vi "Create PINGREQ Packet.vi"(5 "PINGREC in":refnum<class "PINGREC.lvclass">, 8 "error in (no error)":errorcluster) -> (0 "error out":errorcluster, 3 "PINGREC out":refnum<class "PINGREC.lvclass">)   [LabVIEW 2013, in "PINGREC.lvclass"]
uses:
  PINGREC.lvclass
  ControlPacket/ControlPacket.lvclass/ControlPacket.ctl
  ControlPacket/ControlPacket.lvclass
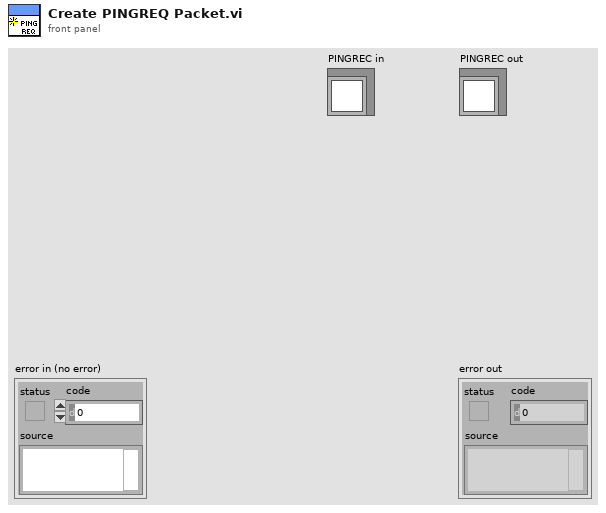
[diagram p1: front panel]
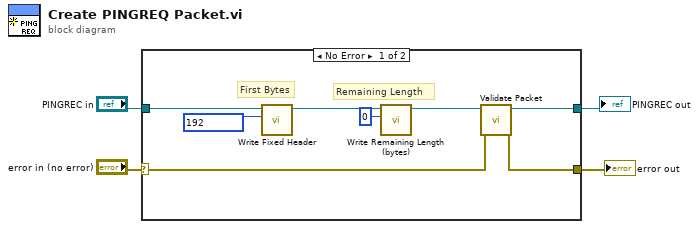
[diagram p0: block diagram]
diagram:
  n1 = case shown="No Error" "error in (no error)" {
    selector: "error in (no error)" -> [w6 w14]
    tunnel: [w5 w14] -> w1
    tunnel: [w7 w13] -> w2
    tunnel: "PINGREC in" -> [w12 w13]
    frame No Error {
      # "Remaining Length"
      # "First Bytes"
      n2 = call "Write Fixed Header.vi"("Fixed Header"=u8 192, "ControlPacket in"=w12) -> ("ControlPacket out"=w11:refnum<class "PINGREC.lvclass">)  [unwired: 9 in]
      n3 = call "Write Remaining Length (bytes).vi"("Remaining Length (bytes)"=u32 0, "ControlPacket in"=w11) -> ("ControlPacket out"=w8:refnum<class "PINGREC.lvclass">)  [unwired: 9 in]
      n4 = call "Validate Packet.vi"("error in (no error)"=w6, "ControlPacket in"=w8) -> ("error out"=w5:errorcluster, "ControlPacket out"=w7:refnum<class "PINGREC.lvclass">)  [unwired: 8 in]
    }
    frame Error {
    }
  }
  "error out" <- w1
  "PINGREC out" <- w2
